vi "Read Write Script 3.vi"(6 "chip select (0)":u32, 8 "error in (no error)":errorcluster, 9 "Write Data":u8[](array[numeric]), 10 "delay in milliseconds (0)":u8, 11 "spi script reference in":T1) -> (0 "error out":errorcluster, 2 "script read index":u32, 3 "spi script reference out":T1)   [LabVIEW 2013]
uses:
  <vilib>/ni845x/ni845x.llb/ni845xSpiScriptControl.ctl
  <vilib>/ni845x/ni845x.llb/NI-845x SPI Script Ms Delay.vi
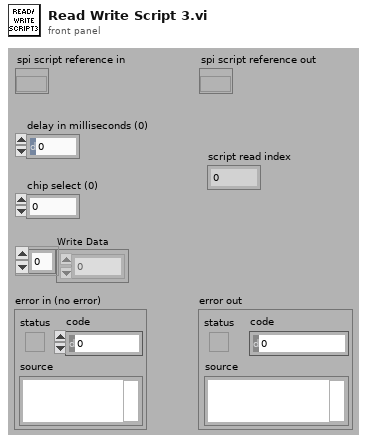
[diagram p1: front panel]
types:
  T1 = typedef "ni845xSpiScriptControl.ctl" = refnum<k20>
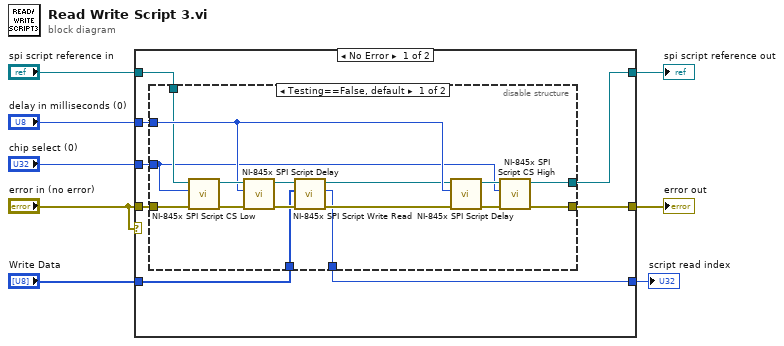
[diagram p0: block diagram]
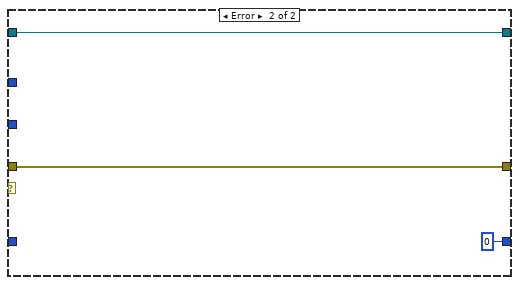
[diagram p3: hidden frame]
diagram:
  n1 = case shown="No Error" "error in (no error)" {
    tunnel: [w9 u32 0 ("script read index")] -> w1
    tunnel: [w16 w36] -> w8
    tunnel: [w15 w37] -> w7
    tunnel: "Write Data" -> [w14 _]
    tunnel: "delay in milliseconds (0)" -> [w13 _]
    tunnel: "error in (no error)" -> [w12 w37]
    tunnel: "spi script reference in" -> [w11 w36]
    tunnel: "chip select (0)" -> [w10 _]
    frame No Error {
      n2 = disable-structure shown="Testing==False, default" {
        disable-tunnel: [w28 w33] -> w16
        disable-tunnel: [w27 w34] -> w15
        disable-tunnel: w14 -> [w20 _]
        disable-tunnel: w13 -> [w26 _]
        disable-tunnel: w12 -> [w25 w34]
        disable-tunnel: w11 -> [w24 w33]
        disable-tunnel: w10 -> [w23 _]
        disable-tunnel: [w17 _] -> w9
        frame condition #0 (active) {
          n3 = call <vilib>:"NI-845x SPI Script CS Low.vi"("error in (no error)"=w25, "chip select (0)"=w23, "spi script reference in"=w24) -> ("error out"=w29:errorcluster, "spi script reference out"=w30:T1)  [unwired: 7 in]
          n4 = call-poly <vilib>:"NI-845x SPI Script Delay.vi"("error in (no error)"=w29, "delay in milliseconds (0)"=w26, "spi script reference in"=w30) -> ("error out"=w21:errorcluster, "spi script reference out"=w22:T1)  [unwired: 7 in]
          n5 = call <vilib>:"NI-845x SPI Script Write Read.vi"("error in (no error)"=w21, "write data"=w20, "spi script reference in"=w22) -> ("error out"=w18:errorcluster, "script read index"=w17:u32, "spi script reference out"=w19:T1)  [unwired: 6 in]
          n6 = call-poly <vilib>:"NI-845x SPI Script Delay.vi"("error in (no error)"=w18, "delay in milliseconds (0)"=w26, "spi script reference in"=w19) -> ("error out"=w31:errorcluster, "spi script reference out"=w32:T1)  [unwired: 7 in]
          n7 = call <vilib>:"NI-845x SPI Script CS High.vi"("error in (no error)"=w31, "chip select (0)"=w23, "spi script reference in"=w32) -> ("error out"=w27:errorcluster, "spi script reference out"=w28:T1)  [unwired: 7 in]
        }
        frame condition #1 {
        }
      }
    }
    frame Error {
    }
  }
  "spi script reference out" <- w8
  "error out" <- w7
  "script read index" <- w1
